vi "IPG RSSI MEASUREMENT.vi"(0 "MICS Resource Name":refnum<visa-resource-name>, 1 "Channel (for RSSI Measurement)":u8=255, 2 "2.45 GHz Power":i8(ring)=6 items=["-29"=-29, "-4"=-4, "-2"=-2, "0"=0, "2"=2, "4"=4, "6"=6, "8"=8, "10"=10, "12"=12, "14"=14, "16"=16, "18"=18, "20"=20, "22"=22, "24"=24, "26"=26, "27"=27], 5 "Delay (for RSSI Measurement)":u16=100, 9 "Duration (for RSSI Measurement)":u16=100, 11 "error in":errorcluster, 12 "MICS Power Setting":u8=28 format="%.0x", 13 "Attenuation dB":dbl) -> (3 "RSSI Values (String, HEX)":string[](array[string]), 4 "MICS Resource Name out":refnum<visa-resource-name>, 6 "RSSI Values":u32[](array[numeric]), 8 "MEAN RSSI":dbl=nan, 10 "MAX RSSI":u32, 14 "MIN RSSI":u32, 15 "error out":errorcluster)   [LabVIEW 2010]
doc: "This function performs an RSSI measurement on the IPG."
uses:
  <vilib>/Analysis/NI_AALBase.lvlib
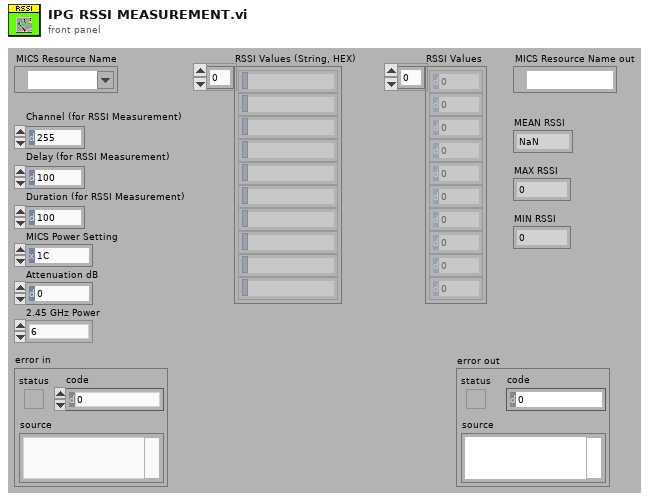
[diagram p1: front panel]
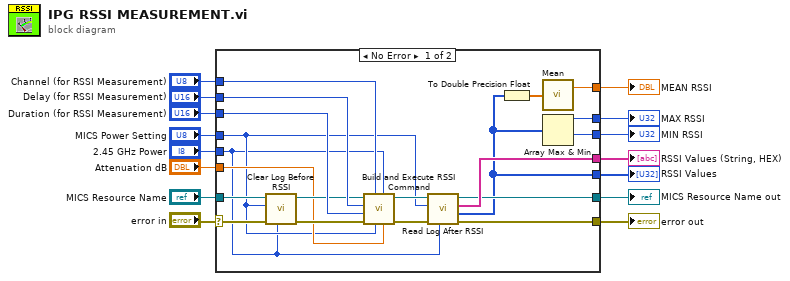
[diagram p0: block diagram]
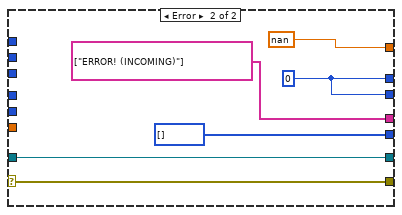
[diagram p2: hidden frame]
diagram:
  n1 = case shown="No Error" "error in" {
    selector: "error in" -> [w31 w41]
    tunnel: [w27 w41] -> w14
    tunnel: [w26 string[] ["ERROR! (INCOMING)"] ("RSSI Values (String)")] -> w13
    tunnel: [w20 u32[] [] ("RSSI Values")] -> w12
    tunnel: [w25 w38] -> w11
    tunnel: "MICS Resource Name" -> [w30 w38]
    tunnel: "Channel (for RSSI Measurement)" -> [w35 _]
    tunnel: "Delay (for RSSI Measurement)" -> [w34 _]
    tunnel: "Duration (for RSSI Measurement)" -> [w33 _]
    tunnel: "MICS Power Setting" -> [w22 _]
    tunnel: "Attenuation dB" -> [w28 _]
    tunnel: "2.45 GHz Power" -> [w16 _]
    tunnel: [w19 nan ("mean")] -> w1
    tunnel: [w18 w36] -> w2
    tunnel: [w17 w36] -> w3
    frame No Error {
      n2 = call "Clear Log Before RSSI.vi"("2.45 GHz Wake-Up Power"=w16, "error in"=w31, "400 MHz MICS Power Setting"=w22, "VISA Resource Name"=w30) -> ("error out"=w32:errorcluster, "dup VISA Resource Name"=w29:refnum<visa-resource-name>)  [unwired: 6 in]
      n3 = call "Build and Execute RSSI Command.vi"("Attenuation dB"=w28, "2.45 GHz Wake-Up Power"=w16, "400 MHz MICS Power Setting"=w22, "Channel (for RSSI Measurement)"=w35, "error in"=w32, "Duration (for RSSI Measurement)"=w33, "Delay (for RSSI Measurement)"=w34, "VISA resource in"=w29) -> ("error out"=w24:errorcluster, "dup VISA resource"=w23:refnum<visa-resource-name>)  [unwired: 2 in]
      n4 = call "Read Log After RSSI.vi"("2.45 GHz Wake-Up Power"=w16, "error in"=w24, "400 MHz MICS Power Setting"=w22, "VISA resource name"=w23) -> ("error out"=w27:errorcluster, "RSSI Values"=w20:u32[], "RSSI Values (String, HEX)"=w26:string[], "dup VISA Resource Name"=w25:refnum<visa-resource-name>)  [unwired: 4 in]
      n5 = To Double Precision Float(number=w20) -> (double precision float=w21:dbl[])
      n6 = call <vilib>:"Mean.vi"("X"=w21) -> ("mean"=w19:dbl)  [unwired: 1 out]
      n7 = Array Max & Min(array=w20) -> (max value=w17:u32, min value=w18:u32)  [unwired: 2 out]
    }
    frame Error {
      w36 = u32 0
    }
  }
  "error out" <- w14
  "RSSI Values (String, HEX)" <- w13
  "RSSI Values" <- w12
  "MICS Resource Name out" <- w11
  "MAX RSSI" <- w3
  "MIN RSSI" <- w2
  "MEAN RSSI" <- w1
